vi "ADS1X15 Example.vi"() -> ()   [LabVIEW 2020]
uses:
  LINX-ADS1015/Channel Selection.ctl
  LINX-ADS1015/ADC Type Selection.ctl
  LINX-ADS1015/ADS1015 Sample Rate.ctl
  LINX-ADS1015/Programmable Gain Selection.ctl
  <vilib>/MakerHub/LINX/Public/Utilities/Open Local.vi
  LINX I2C/LINX I2C.lvclass
  LINX-ADS1015/LINX-ADS1X15.lvclass
  <vilib>/MakerHub/LINX/LMH-LINX.lvlib
panel:
  in  "Channels":T1[](array[typedef])=[16384] items=["Differential 0-1"=0, "Differential 2-3"=12288, "Single Ended 0"=16384, "Single Ended 1"=20480, "Single Ended 2"=24576, "Single Ended 3"=28672]
  out "Waveform Chart":dbl[][](graph)
  in  "stop":bool
  out "Error Out":errorcluster
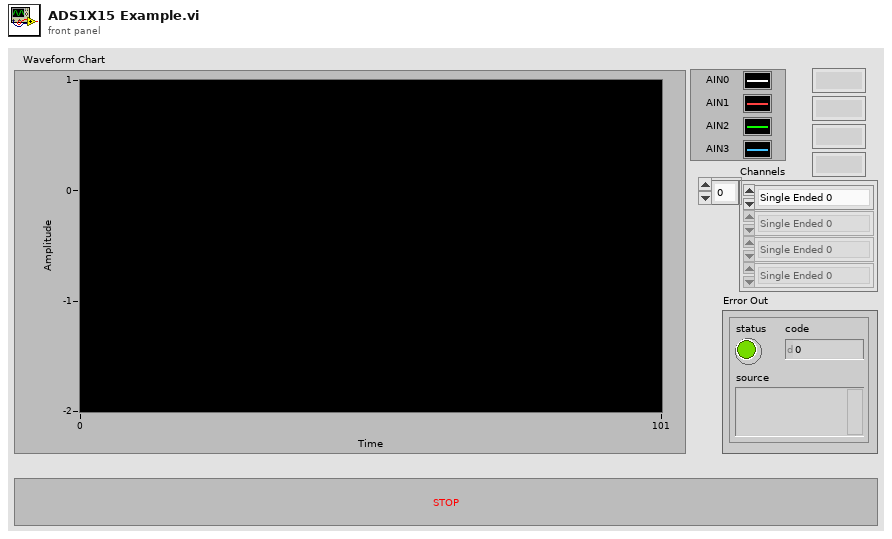
[diagram p1: front panel]
types:
  T1 = typedef "LINX-ADS1X15.lvclass/Channel Selection.ctl" = u16
  T2 = typedef "LINX-ADS1X15.lvclass/Programmable Gain Selection.ctl" = u16
  T3 = typedef "LINX-ADS1X15.lvclass/ADS1015 Sample Rate.ctl" = u16
  T4 = typedef "LINX-ADS1X15.lvclass/ADC Type Selection.ctl" = enum16{"ADS1015", "ADS1115"}
  T5 = typedef "LMH-LINX.lvlib/LINX Ref.ctl" = cluster{"IO":T6, "Interface":T7, "LINX Device Config":T8}
  T6 = typedef "LMH-LINX.lvlib/Platform.ctl" = enum16{"Remote", "Local"}
  T7 = typedef "LMH-LINX.lvlib/Interface.ctl" = enum16{"Serial", "TCP"}
  T8 = typedef "LMH-LINX.lvlib/Device.lvlib/LINX Device Config.ctl" = cluster{"Interface":T7, "COM Port":refnum<visa-resource-name>, "TCP Configuration":T9, "Device Family":u8, "Device ID":u8, "Device Name":string, "TCP Ref":refnum<k5>, "Channels":T10}
  T9 = typedef "LMH-LINX.lvlib/Device.lvlib/TCP Config.ctl" = cluster{"IP Address":string, "Port":u16}
  T10 = typedef "LMH-LINX.lvlib/Channels.ctl" = cluster{"DI":u8[], "DO":u8[], "AI":u8[], "AO":u8[], "PWM":u8[], "QE":u8[], "UART":u8[], "I2C 2":u8[], "SPI":u8[], "CAN":u8[], "Servo":u8[], "AI Ref (V)":dbl, "AI Resolution (Bits)":u8, "AO Ref (V)":dbl, "AO Resolution (Bits)":u8}
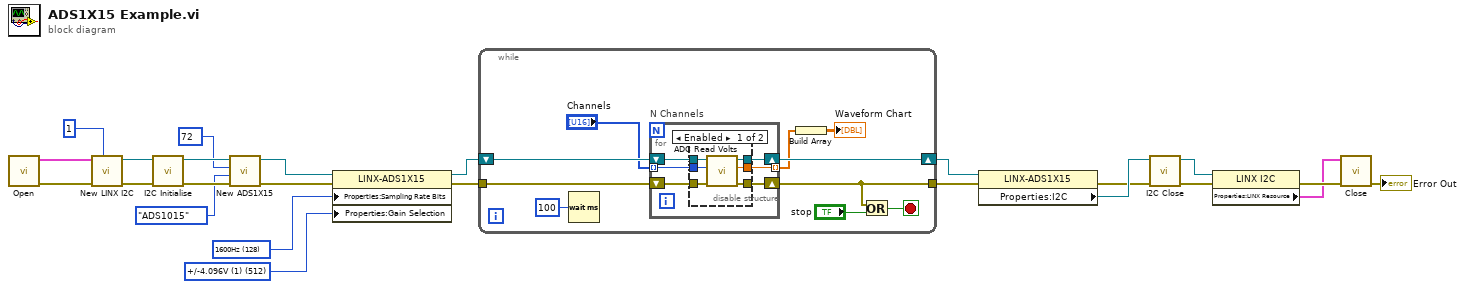
[diagram p0: block diagram]
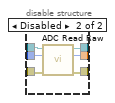
[diagram p2: hidden frame]
diagram:
  w3 = T2 512 items=["+/-6.144V (2/3)"=0, "+/-4.096V (1)"=512, "+/-2.048V (2)"=1024, "+/-1.024V (4)"=1536, "+/-0.512V (8)"=2048, "+/-0.256V (16)"=2560] ("Gain Selection")
  w4 = T3 128 items=["128Hz"=0, "250Hz"=32, "490Hz"=64, "920Hz"=96, "1600Hz"=128, "2400Hz"=160, "3300Hz"=192] ("ADS1015 Sample Rate")
  n1 = call-poly <vilib>:"Open.vi"() -> ("Error Out"=w22:errorcluster, "LINX Resource"=w23:T5)  [unwired: 9 in, 1 out]
  n2 = call "New LINX I2C.vi"("LINX I2C Channel"=u8 1 ("I2C Channel"), "error in (no error)"=w22, "LINX Resource"=w23) -> ("error out"=w20:errorcluster, "LINX I2C out"=w19:refnum<class "LINX I2C.lvclass">)  [unwired: 7 in]
  n3 = call-dynamic "I2C Initialise.vi"("error in (no error)"=w20, "LINX I2C in"=w19) -> ("error out"=w12:errorcluster, "LINX I2C out"=w11:refnum<class "LINX I2C.lvclass">)  [unwired: 8 in]
  n4 = call "New ADS1X15.vi"("error in (no error)"=w12, "ADC Type (ADS1015)"=ADC_Type_Selection."ADS1015", "I2C Slave Address (0x48)"=u8 72, "I2C"=w11) -> ("error out"=w6:errorcluster, "LINX-ADS1X15 out"=w9:refnum<class "LINX-ADS1X15.lvclass">)  [unwired: 6 in]
  n5 = property class="LINX-ADS1X15"(reference=w9, error in=w6, "Properties:Sampling Rate Bits"=w4, "Properties:Gain Selection"=w3) -> (reference out=w7:refnum<class "LINX-ADS1X15.lvclass">, error out=w5:errorcluster)
  n6 = while {
    tunnel: w5 -> [w33]
    shift-right: [w29] -> w2
    shift-left: w7 -> [w34]
    tunnel: [w28] -> w1
    stop <- w30 stop-if-true
    n7 = Wait (ms)(milliseconds to wait=u32 100) -> ()  [unwired: 1 out]
    n8 = for "N Channels" {
      tunnel: "Channels" -> [w38] mode=indexing
      tunnel: [w35] -> w27 mode=indexing
      shift-right: [w37] -> w29
      shift-left: w34 -> [w40]
      shift-right: [w36] -> w28
      shift-left: w33 -> [w39]
      n9 = disable-structure shown="Enabled" {
        disable-tunnel: w40 -> [w46 w52]
        disable-tunnel: w39 -> [w45 w51]
        disable-tunnel: w38 -> [w44 w50]
        disable-tunnel: [w43 w49] -> w37
        disable-tunnel: [w42 w47] -> w36
        disable-tunnel: [w41 w48] -> w35
        frame Enabled {
          n10 = call "ADC Read Volts.vi"("error in (no error)"=w45, "ADC Channel Selection"=w44, "LINX-ADS1X15 in"=w46) -> ("error out"=w42:errorcluster, "ADC Volts"=w41:dbl, "LINX-ADS1X15 out"=w43:refnum<class "LINX-ADS1X15.lvclass">)  [unwired: 6 in]
        }
        frame Disabled {
          n11 = call-dynamic "ADC Read Raw.vi"("error in (no error)"=w51, "ADC Channel Selection"=w50, "LINX-ADS1X15 in"=w52) -> ("error out"=w47:errorcluster, "ADC Raw"=w48:i16, "LINX-ADS1X15 out"=w49:refnum<class "LINX-ADS1X15.lvclass">)  [unwired: 6 in]
        }
      }
    }
    n12 = Build Array(w27) -> (→"Waveform Chart":dbl[][])
    n13 = Or(x=w28, y="stop") -> (x .or. y?=w30:bool)
  }
  n14 = property class="LINX-ADS1X15"(reference=w2, error in=w1) -> (error out=w17:errorcluster, "Properties:I2C"=w18:refnum<class "LINX I2C.lvclass">)  [unwired: 1 out]
  n15 = call-dynamic "I2C Close.vi"("error in (no error)"=w17, "LINX I2C in"=w18) -> ("error out"=w16:errorcluster, "LINX I2C out"=w14:refnum<class "LINX I2C.lvclass">)  [unwired: 8 in]
  n16 = property class="LINX I2C"(reference=w14, error in=w16) -> (error out=w15:errorcluster, "Properties:LINX Resource"=w13:T5)  [unwired: 1 out]
  n17 = call <vilib>:"Close.vi"("Error In"=w15, "LINX Resource"=w13) -> ("Error Out"=→"Error Out":errorcluster)  [unwired: 9 in]
